vi "Open Sender UDP Connection.vi"(5 "Local Port":i32=3455) -> (0 "error out":errorcluster, 2 "UDP Network Connection Refnum":refnum<k16>)   [LabVIEW 2013]
uses:
  subVIs.llb/UDP Multicast Open.vi
panel:
  in  "TTL":u16=1
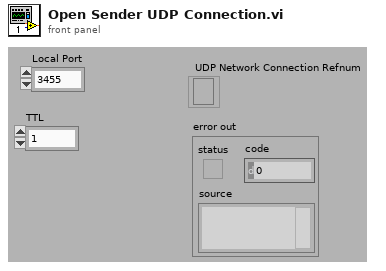
[diagram p1: front panel]
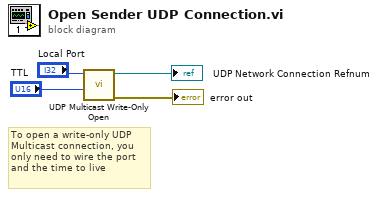
[diagram p0: block diagram]
diagram:
  # "To open a write-only UDP\nMulticast connection, you\nonly need to wire the port\nand the time to live"
  n1 = call-poly "UDP Multicast Write-Only Open.vi"("time-to-live (1)"="TTL", "port"="Local Port") -> ("error out"=→"error out":errorcluster, "connection ID"=→"UDP Network Connection Refnum":refnum<k16>)  [unwired: 1 in, 7 out]
